vi "util-address-parser.vi"(10 "ADDR 2":T1 format="%04d") -> (1 "Channel":u8 format="%02d", 2 "Address":u8 format="%02d")   [LabVIEW 2024]
uses:
  controls/type.address.ctl
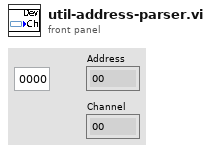
[diagram p1: front panel]
types:
  T1 = typedef "type.address.ctl" = u16
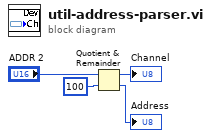
[diagram p0: block diagram]
diagram:
  n1 = Quotient & Remainder(x="ADDR 2", y=u16 100) -> (x-y*floor(x/y)=→"Channel":T1, floor(x/y)=→"Address":T1)
